vi "Init.vi"(7 "Process Name":string, 8 "error in (no error)":errorcluster) -> (0 "error out":errorcluster)   [LabVIEW 2016, in "System.lvlib"]
uses:
  System.lvlib
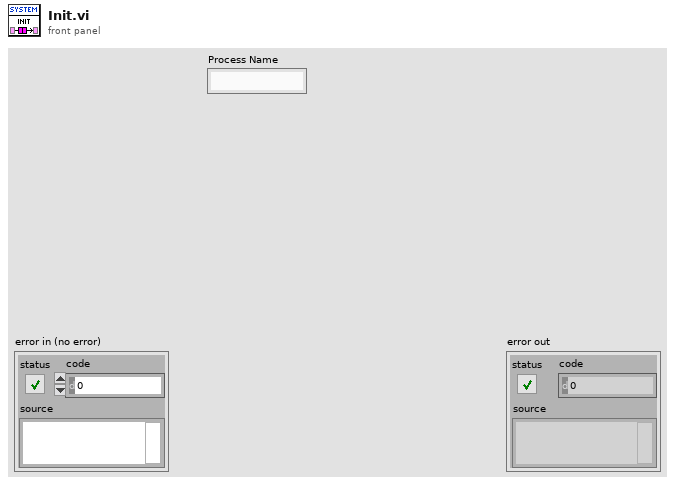
[diagram p1: front panel]
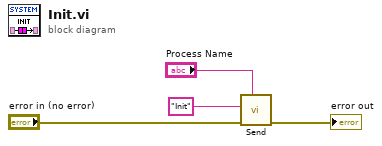
[diagram p0: block diagram]
diagram:
  n1 = call "Send.vi"("Process Name"="Process Name", "error in (no error)"="error in (no error)", "Message"="Init") -> ("error out"=→"error out":errorcluster)  [unwired: 8 in]
